vi "Team Move.vi"(6 "MIA[]":T1[](array[typedef]), 8 "error in (no error)":errorcluster, 9 "Info in[Player]":T1[](array[typedef]), 10 "p[x][y]":i32[][](array[numeric]), 11 "TeamEffort in":refnum<class "TeamEffort.lvclass">) -> (0 "error out":errorcluster, 1 "Info out[Player]":T2[](array[typedef]), 3 "TeamEffort out":refnum<class "TeamEffort.lvclass">)   [LabVIEW 2015, in "TeamEffort.lvclass"]
uses:
  TeamEffort.lvclass
  Team Move Output.ctl
  Square/Square.lvclass
  Type Defs/Action Enum.ctl
  Type Defs/Direction Enum.ctl
  Team Move Input.ctl
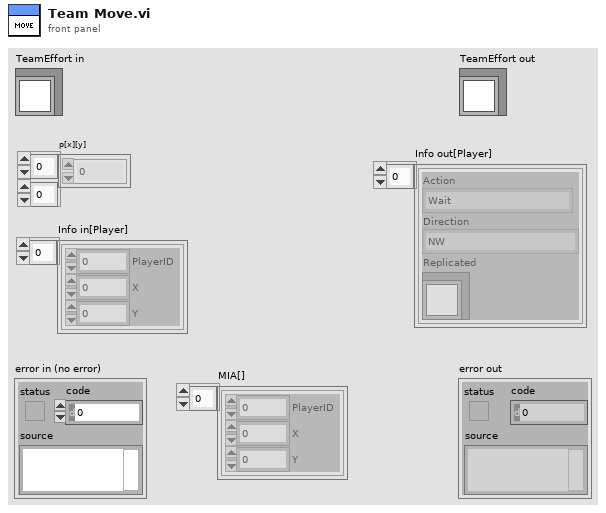
[diagram p1: front panel]
types:
  T1 = typedef "TeamEffort.lvclass/Team Move Input.ctl" = cluster{"PlayerID":i32, "X":i32, "Y":i32}
  T2 = typedef "TeamEffort.lvclass/Team Move Output.ctl" = cluster{"Action":T3, "Direction":T4, "Replicated":refnum<class "Square.lvclass">}
  T3 = typedef "Square.lvclass/Action Enum.ctl" = enum16{"Wait", "Move", "Attack", "Replicate"}
  T4 = typedef "Square.lvclass/Direction Enum.ctl" = enum16{"NW", "N", "NE", "E", "SE", "S", "SW", "W"}
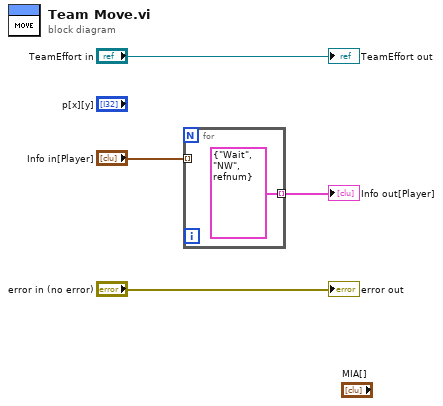
[diagram p0: block diagram]
diagram:
  n1 = for {
    tunnel: "Info in[Player]" -> [_] mode=indexing
    tunnel: [T2 {"Action"=enum."Wait", "Direction"=enum."NW", "Replicated"=refnum} ("Cluster")] -> w1 mode=indexing
  }
  "Info out[Player]" <- w1
  "error out" <- "error in (no error)"
  "TeamEffort out" <- "TeamEffort in"
